vi "Calculate Wavelength.vi"(8 "error in (no error)":errorcluster, 9 "Offset in Wavlength (nm)":dbl=10.0 min=0.0 max=100.0, 10 "Number of Pixels (3648)":i32=3648, 11 "VISA resource name":refnum<visa-resource-name>) -> (0 "error out":errorcluster, 2 "Wavelength (nm)":dbl[](array[numeric]), 3 "VISA resource name out":refnum<visa-resource-name>)   [LabVIEW 2013, in "Ocean Optics 2000 4000.lvlib"]
doc: "Calculate the wavelength from each pixel number."
uses:
  <instrlib>/Ocean Optics 2000 4000/Ocean Optics 2000 4000.lvlib
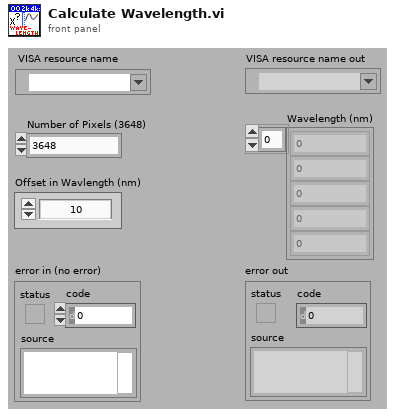
[diagram p1: front panel]
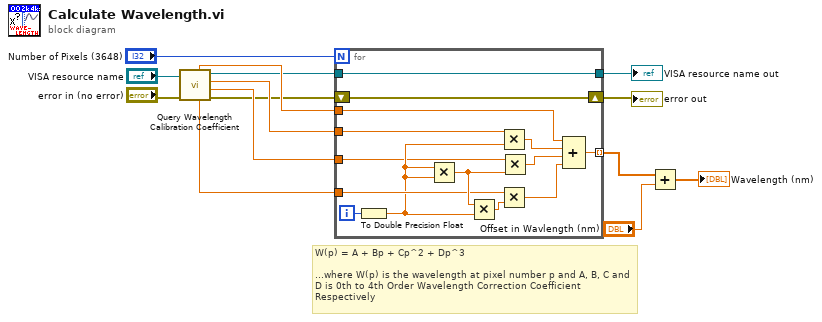
[diagram p0: block diagram]
diagram:
  # "W(p) = A + Bp + Cp^2 + Dp^3  \n\n...where W(p) is the wavelength at pixel number p and A, B, C and D is 0th to 4th Order Wavelength Correction Coefficient Respectively"
  n1 = call <instrlib>:"Query Wavelength Calibration Coefficient.vi"("error in (no error)"="error in (no error)", "VISA resource name"="VISA resource name") -> ("error out"=w7:errorcluster, "2nd Order Wavelength Calibration Coefficient"=w10:dbl, "1st Order Wavelength Calibration Coefficient"=w11:dbl, "VISA resource name out"=w8:refnum<visa-resource-name>, "3rd Order Wavelength Calibration Coefficient"=w9:dbl, "0th Order Wavelength Calibration Coefficient"=w12:dbl)  [unwired: 4 in]
  n2 = for {
    N: "Number of Pixels (3648)" -> [_]
    tunnel: w11 -> [w28]
    tunnel: w12 -> [w23]
    tunnel: w9 -> [w21]
    tunnel: [w18] -> w3 mode=indexing
    tunnel: w10 -> [w17]
    tunnel: w8 -> [w16]
    tunnel: [w16] -> w6
    shift-right: [w15] -> w5
    shift-left: w7 -> [w15]
    i -> [w24]
    n3 = To Double Precision Float(number=w24) -> (double precision float=w19:dbl)
    n4 = Multiply(x=w19, y=w19) -> (x*y=w25:dbl)
    n5 = Multiply(x=w25, y=w19) -> (x*y=w22:dbl)
    n6 = Multiply(x=w28, y=w19) -> (x*y=w26:dbl)
    n7 = Multiply(x=w21, y=w22) -> (x*y=w20:dbl)
    n8 = Multiply(x=w17, y=w25) -> (x*y=w27:dbl)
    n9 = Compound Arithmetic op=ADD(w23, w26, w27, w20) -> (w18:dbl)
  }
  "VISA resource name out" <- w6
  "error out" <- w5
  n10 = Add(x=w3, y="Offset in Wavlength (nm)") -> (x+y=→"Wavelength (nm)":dbl[])
